vi "CAN_STOP.vi"(3 "error in":errorcluster, 5 "CANopen Session In":refnum<class "sbCANopenBaseClass.lvclass">) -> (0 "error out":errorcluster)   [LabVIEW 2024]
uses:
  <vilib>/addons/Maxon Motor/EPOS2 CANopen/CANopen/sbCANopenBaseClass.lvclass
  <vilib>/addons/Maxon Motor/EPOS2 CANopen/EPOS2 Library.lvlib
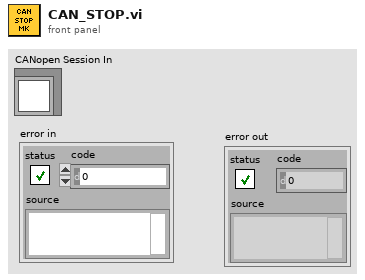
[diagram p1: front panel]
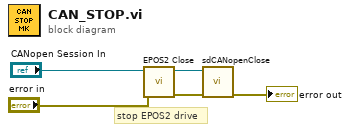
[diagram p0: block diagram]
diagram:
  # "stop EPOS2 drive"
  n1 = call <vilib>:"EPOS2 Close.vi"("error in"="error in", "CANopen Session In"="CANopen Session In") -> ("error out"=w4:errorcluster, "CANopen Session Out"=w5:refnum<class "sbCANopenBaseClass.lvclass">)  [unwired: 2 in, 6 out]
  n2 = call-dynamic "sdCANopenClose.vi"("error in (no error)"=w4, "sbCANopenBaseClass in"=w5) -> ("error out"=→"error out":errorcluster)  [unwired: 8 in, 1 out]
